vi "Set Scaling Strategy.vi"(10 "Scaling Strategy":refnum<class "Scaling Strategy.lvclass">, 11 "Virtual Instrument in":refnum<class "Virtual Instrument.lvclass">) -> (3 "Virtual Instrument out":refnum<class "Virtual Instrument.lvclass">)   [LabVIEW 2024, in "HAL.lvlib" / "Virtual Instrument.lvclass"]
uses:
  Virtual Instrument.lvclass
  Scaling Strategy/Scaling Strategy.lvclass
  Virtual Instrument.lvclass/Virtual Instrument.ctl
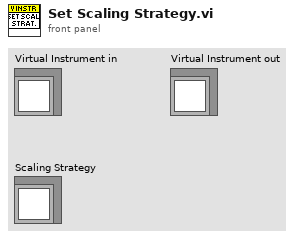
[diagram p1: front panel]
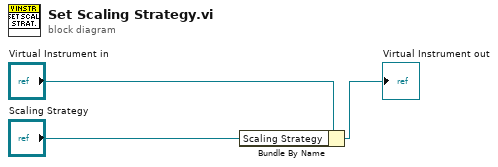
[diagram p0: block diagram]
diagram:
  n1 = Bundle By Name(cluster="Virtual Instrument in", "Scaling Strategy"="Scaling Strategy") -> (→"Virtual Instrument out":refnum<class "Virtual Instrument.lvclass">)
